vi "FGV_Terminal.vi"() -> ()   [LabVIEW 2014]
uses:
  TerminalAction.ctl
panel:
  in  "Action":T1=enum."Add Item"
  in  "Terminaln":string
  out "TerminalOut":string
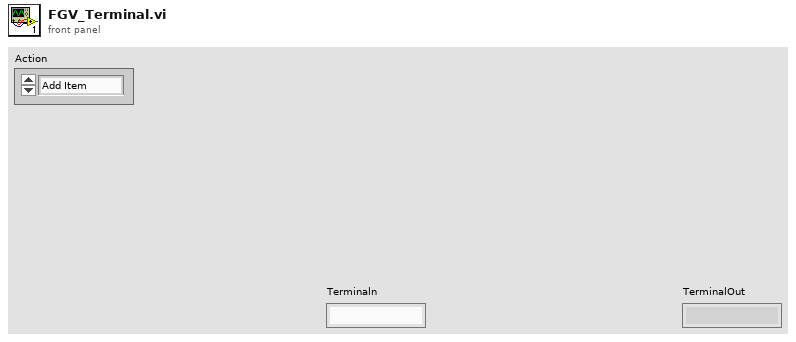
[diagram p1: front panel]
types:
  T1 = typedef "TerminalAction.ctl" = enum16{"Get Terminal", "Set Terminal", "Add Item", "Clear Terminal"}
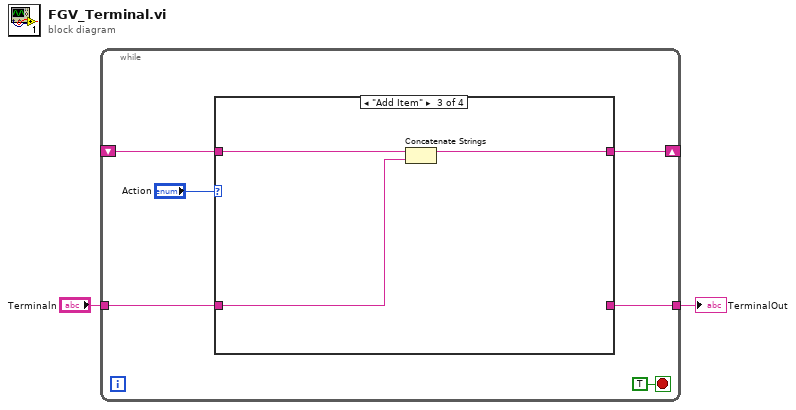
[diagram p0: block diagram]
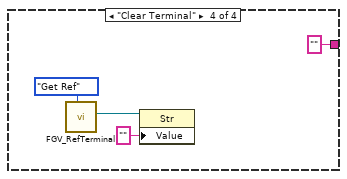
[diagram p4: hidden frame]
diagram:
  n1 = while {
    tunnel: "Terminaln" -> [w7]
    shift-right: [w6] -> _
    shift-left: _ -> [w4]
    tunnel: [w5] -> w1
    stop <- TRUE stop-if-true
    n2 = case shown="\"Add Item\"" "Action" {
      tunnel: w7 -> [_ w10 w13 _]
      tunnel: [w9 w10 w11 "" ("Terminaln")] -> w6
      tunnel: [w9 _ _ _] -> w5
      tunnel: w4 -> [w9 _ w12 _]
      frame "Get Terminal", Default {
      }
      frame "Set Terminal" {
      }
      frame "Add Item" {
        n3 = Concatenate Strings(w12, w13) -> (w11:string)
      }
      frame "Clear Terminal" {
        n4 = call "FGV_RefTerminal.vi"("Action"=enum16{"Set Ref", "Get Ref"}."Get Ref") -> ("refout"=w15:refnum<vi>)  [unwired: 10 in]
        n5 = property class="Str"(reference=w15, "Value"="") -> ()  [unwired: 1 in, 2 out]
      }
    }
  }
  "TerminalOut" <- w1
